vi "Get 2D Time Stamp.vi"(5 "format string (%s)":string="%s", 7 "key description":string, 8 "sections":string[](array[string]), 9 "time stamp":timestamp[][](array[timestamp]), 11 "info data":string) -> (0 "sections out":string[](array[string]), 2 "value":timestamp[][](array[timestamp]), 3 "info data out":string)   [LabVIEW 2019, in "infolib.lvlib"]
doc: "Reads matrix of time stamps. If section is entered it searches the key in the section(s)."
uses:
  infolib.lvlib
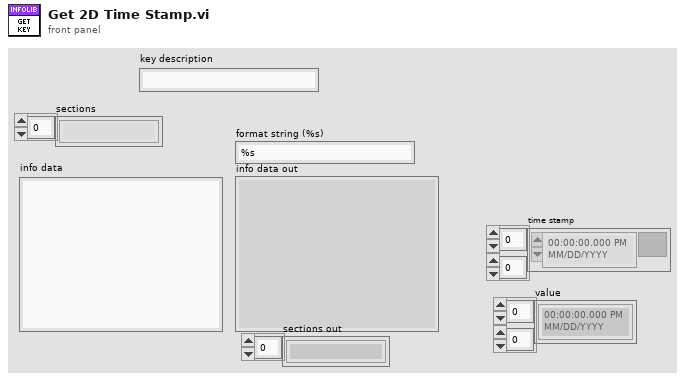
[diagram p1: front panel]
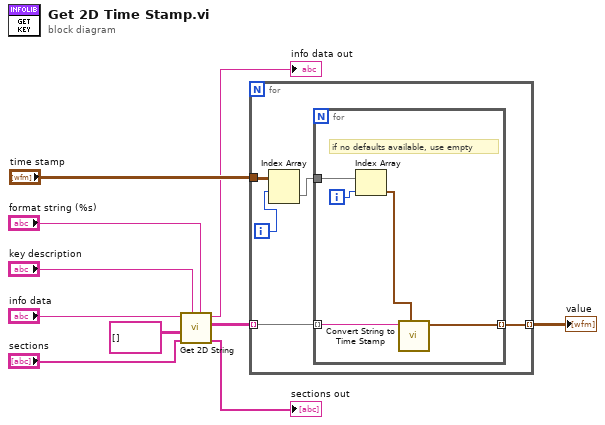
[diagram p0: block diagram]
diagram:
  n1 = call "Get 2D String.vi"("format string (%s)"="format string (%s)", "key description"="key description", "sections"="sections", "string"=string[][] [] ("1D string array"), "info data"="info data") -> ("sections out"=→"sections out":string[], "value"=w1:string[][], "info data out"=→"info data out":string)  [unwired: 4 in]
  n2 = for {
    tunnel: [w15] -> w10 mode=indexing
    tunnel: "time stamp" -> [w13]
    tunnel: w1 -> [w14] mode=indexing
    i -> [w12]
    n3 = Index Array(array=w13, index (row)=w12) -> (element=w11:timestamp[])  [unwired: 1 in]
    n4 = for {
      tunnel: w11 -> [w20]
      tunnel: w14 -> [w19] mode=indexing
      tunnel: [w17] -> w15 mode=indexing
      i -> [w16]
      # "if no defaults available, use empty"
      n5 = Index Array(array=w20, index=w16) -> (element=w18:timestamp)
      n6 = call "Convert String to Time Stamp.vi"("default value of time stamp"=w18, "string"=w19) -> ("time stamp out"=w17:timestamp)  [unwired: 9 in]
    }
  }
  "value" <- w10
